vi "GV_timedToolButtonsUpdate.vi"(8 "error in (no error)":errorcluster, 11 "Gviewer in":refnum<class "Gviewer.lvclass">) -> (0 "error out":errorcluster, 3 "Gviewer out":refnum<class "Gviewer.lvclass">)   [LabVIEW 2020, in "Sgraph_lib_V1.lvlib" / "Gviewer.lvclass"]
doc: "Reset the event timer for the tool buttons update"
uses:
  Gviewer.lvclass
  Gviewer.lvclass/Gviewer.ctl
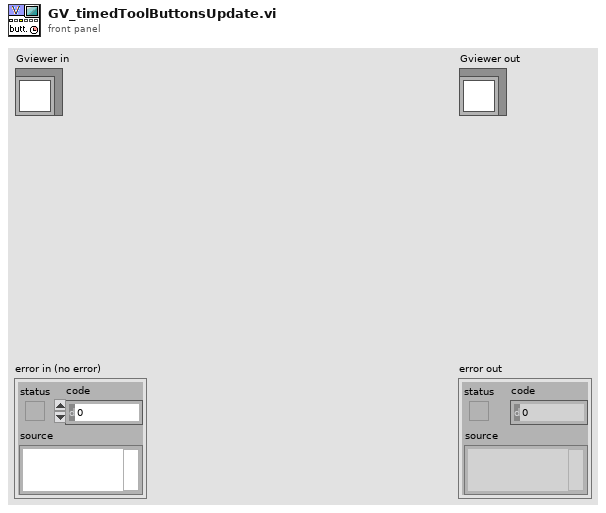
[diagram p1: front panel]
types:
  T1 = typedef "Sgraph_lib_V1.lvlib/Gviewer.lvclass/AttrIdleTimedEvents.ctl" = cluster{"UpdateToolButtons":timestamp, "RedrawGraphUpdate":timestamp, "RequestUpdate":timestamp, "Resize":timestamp}
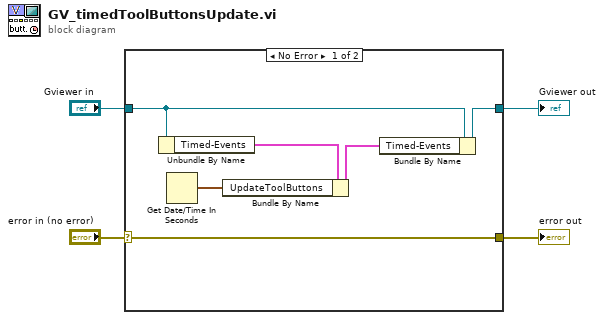
[diagram p0: block diagram]
diagram:
  n1 = case shown="No Error" "error in (no error)" {
    selector: "error in (no error)" -> [w10 w12]
    tunnel: [w10 w12] -> w3
    tunnel: [w9 w11] -> w1
    tunnel: "Gviewer in" -> [w8 w11]
    frame No Error {
      n2 = Unbundle By Name(w8) -> ("Timed-Events"=w7:T1)
      n3 = Get Date/Time In Seconds() -> (seconds since 1Jan1904=w5:timestamp)
      n4 = Bundle By Name(cluster=w7, "UpdateToolButtons"=w5) -> (w6:T1)
      n5 = Bundle By Name(cluster=w8, "Timed-Events"=w6) -> (w9:refnum<class "Gviewer.lvclass">)
    }
    frame Error {
    }
  }
  "error out" <- w3
  "Gviewer out" <- w1
